vi "GetVerticalRange(OLD).vi"(8 "error in (no error)":errorcluster, 10 "Channel (0: Channel 1)":u16(ring) items=["Channel 1", "Channel 2", "Channel 3", "Channel 4", "Math", "Reference 1", "Reference 2", "Reference 3", "Reference 4", "Bus 1", "Bus 2"], 11 "VISA Refnum in":refnum<visa-resource-name>) -> (0 "error out":errorcluster, 2 "VerrticalRange":dbl, 3 "VISA Refnum out":refnum<visa-resource-name>)   [LabVIEW 2013]
doc: "Read from the phsyical device the offset relative to the specified channel"
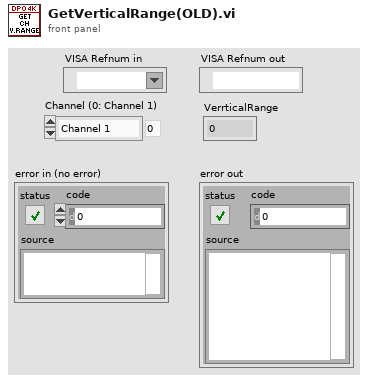
[diagram p1: front panel]
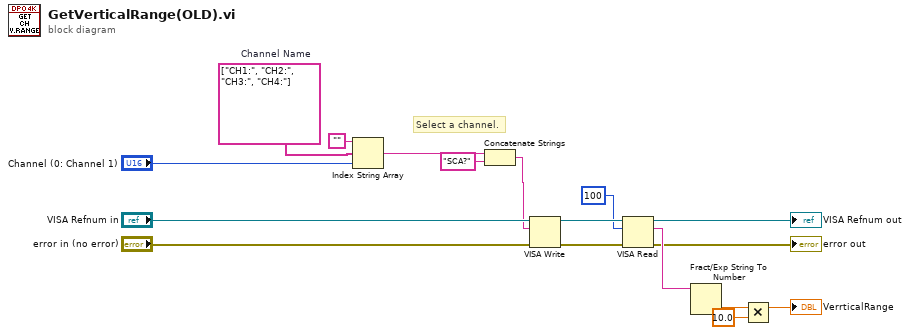
[diagram p0: block diagram]
diagram:
  w8 = string[] ["CH1:", "CH2:", "CH3:", "CH4:"]  # Channel Name
  # "Select a channel."
  n1 = Index String Array(1:"Channel (0: Channel 1)", 2:w8, 3:"") -> (0:w6:string)
  n2 = Concatenate Strings(w6, "SCA?" ("string")) -> (w4:string)
  n3 = VISA Write(VISA resource name="VISA Refnum in", write buffer=w4, error in (no error)="error in (no error)") -> (VISA resource name out=w12:refnum<visa-resource-name>, error out=w10:errorcluster)  [unwired: 1 out]
  n4 = VISA Read(VISA resource name=w12, byte count=u32 100, error in (no error)=w10) -> (VISA resource name out=→"VISA Refnum out":refnum<visa-resource-name>, read buffer=w15:string, error out=→"error out":errorcluster)  [unwired: 1 out]
  n5 = Fract/Exp String To Number(string=w15) -> (number=w3:dbl)  [unwired: 3 in, 1 out]
  n6 = Multiply(x=w3, y=10.0) -> (x*y=→"VerrticalRange":dbl)
